vi "SetPolyInstanceInfo.vi"(2 "InstanceInfo":T1(array[cluster]), 8 "error in (no error)":errorcluster, 11 "Poly VI Path":path) -> (0 "error out":errorcluster)   [LabVIEW 2020]
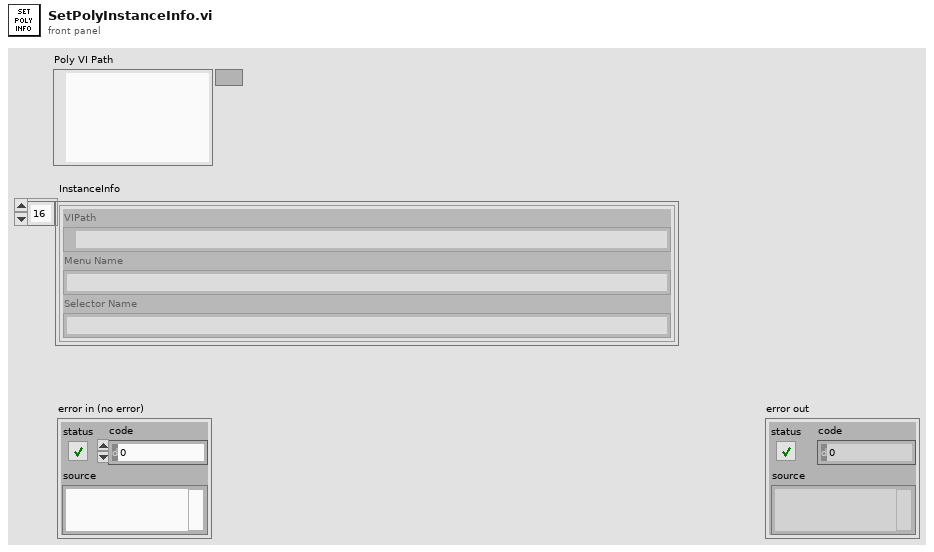
[diagram p1: front panel]
types:
  T1 = cluster{"VIPath":path, "Menu Name":string, "Selector Name":string}[]
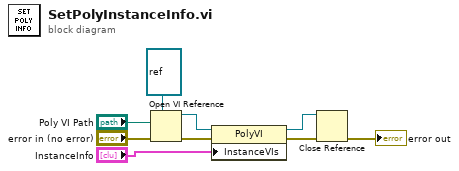
[diagram p0: block diagram]
diagram:
  n1 = Open VI Reference(type specifier VI Refnum (for type only)=refnum<vi> refnum, vi path="Poly VI Path", error in (no error)="error in (no error)") -> (vi reference=w7:refnum<vi>, error out=w6:errorcluster)  [unwired: 3 in]
  n2 = property class="PolyVI"(reference=w7, error in=w6, "InstanceVIs"="InstanceInfo") -> (reference out=w4:refnum<vi>, error out=w5:errorcluster)
  n3 = Close Reference(reference=w4, error in (no error)=w5) -> (error out=→"error out":errorcluster)
